vi "Check pcb cont is connected.vi"(8 "error in (no error)":errorcluster) -> (0 "error out":errorcluster)   [LabVIEW 2016]
uses:
  <vilib>/ULx/Create Channel.llb/ULx Create Channel (DO-Digital Output).vi
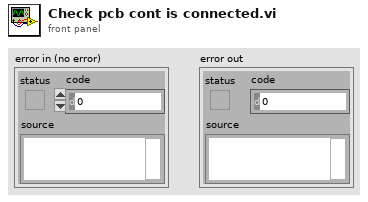
[diagram p1: front panel]
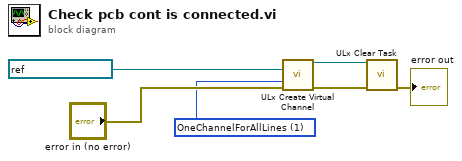
[diagram p0: block diagram]
diagram:
  w1 = 1 items=["OneChannelForEachLine", "OneChannelForAllLines"] ("line grouping")
  n1 = call-poly <vilib>:"ULx Create Virtual Channel.vi"("lines"=refnum<k21> "Dev0/1stPortA" ("Port 2"), "line grouping"=w1, "error in"="error in (no error)") -> ("task out"=w3:refnum<k24>, "error out"=w4:errorcluster)  [unwired: 11 in]
  n2 = call <vilib>:"ULx Clear Task.vi"("task in"=w3, "error in"=w4) -> ("error out"=→"error out":errorcluster)  [unwired: 13 in]
